vi "WRITE.vi"(0 "Z-DATA":path, 1 "Y-DATA":path, 2 "X-DATA":path, 3 "Z":dbl[](array[numeric]), 4 "Y":dbl[](array[numeric]), 5 "X":dbl[](array[numeric])) -> ()   [LabVIEW 2021]
uses:
  <vilib>/Utility/file.llb/Write Delimited Spreadsheet (DBL).vi
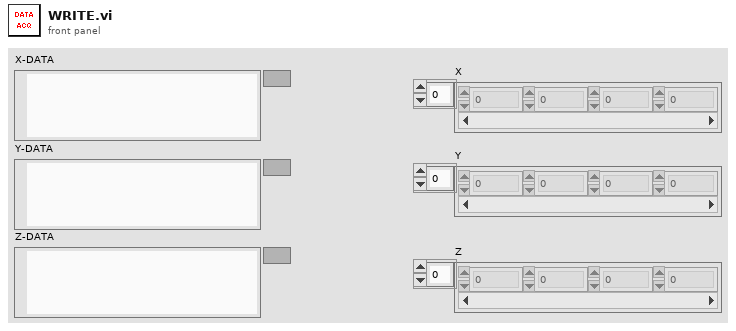
[diagram p1: front panel]
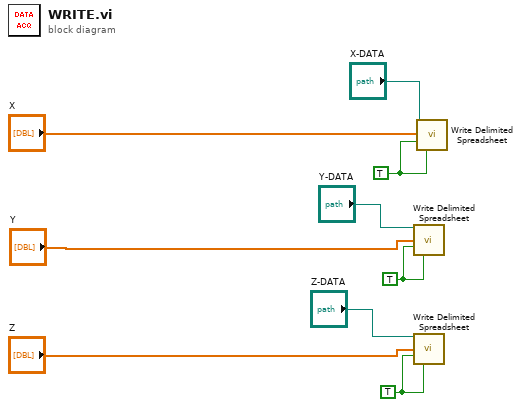
[diagram p0: block diagram]
diagram:
  w1 = TRUE ("append to file? (new file:F)")
  w2 = TRUE ("append to file? (new file:F)")
  w6 = TRUE ("append to file? (new file:F)")
  n1 = call-poly <vilib>:"Write Delimited Spreadsheet.vi"("file path (dialog if empty)"="Y-DATA", "1D data"="Y", "append to file? (new file:F)"=w2, "transpose? (no:F)"=w2) -> ()  [unwired: 10 in, 2 out]
  n2 = call-poly <vilib>:"Write Delimited Spreadsheet.vi"("file path (dialog if empty)"="Z-DATA", "1D data"="Z", "append to file? (new file:F)"=w1, "transpose? (no:F)"=w1) -> ()  [unwired: 10 in, 2 out]
  n3 = call-poly <vilib>:"Write Delimited Spreadsheet.vi"("file path (dialog if empty)"="X-DATA", "1D data"="X", "append to file? (new file:F)"=w6, "transpose? (no:F)"=w6) -> ()  [unwired: 10 in, 2 out]
